vi "Ready Frequency Control for Sync.vi"(8 "error in (no error)":errorcluster, 11 "IED in":refnum<class "IED.lvclass">) -> (0 "error out":errorcluster, 3 "IED out":refnum<class "IED.lvclass">)   [LabVIEW 2015, in "IED Actor.lvlib" / "IED.lvclass"]
uses:
  IED.lvclass
  IED.lvclass/IED.ctl
  <vilib>/NI/Tools/Keyed Array/Map String.vi
  <vilib>/NI/Tools/String/Get Case Matching.vi
  <vilib>/Modbus/master/Modbus Master.lvclass
  <vilib>/NI/Tools/Keyed Array/Tools_KeyedArray.lvlib
  Utilities/Message Strings.llb/Message String Utilities.lvlib
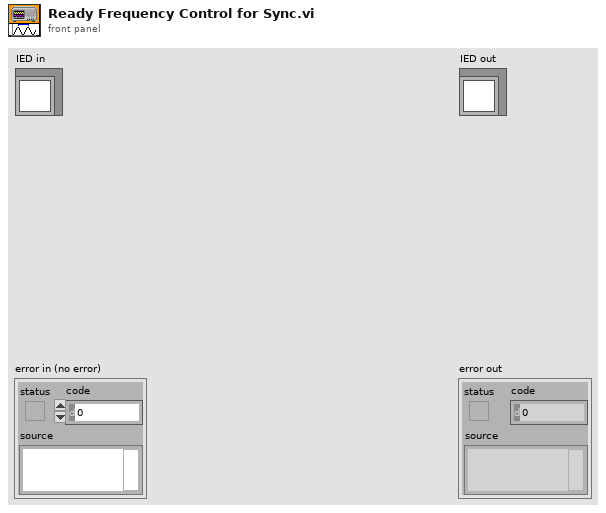
[diagram p1: front panel]
types:
  T1 = typedef "Tools_KeyedArray.lvlib/KeyedArray.ctl" = cluster{"keys":string[], "values":string[]}
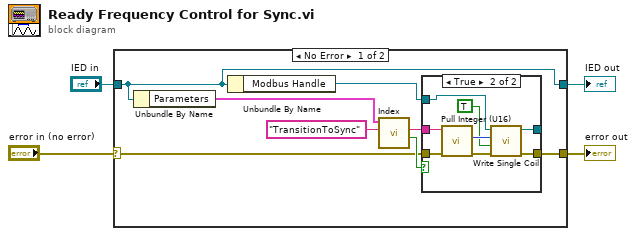
[diagram p0: block diagram]
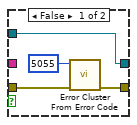
[diagram p2: hidden frame]
diagram:
  n1 = case shown="No Error" "error in (no error)" {
    selector: "error in (no error)" -> [w9 w26]
    tunnel: [w6 w26] -> w3
    tunnel: [w7 w25] -> w1
    tunnel: "IED in" -> [w7 w25]
    frame No Error {
      n2 = Unbundle By Name(w7) -> ("Parameters"=w12:T1)
      n3 = Unbundle By Name(w7) -> ("Modbus Handle"=w8:refnum<class "Modbus Master.lvclass">)
      n4 = call <vilib>:"Index.vi"("key"="TransitionToSync" ("Name"), "array in"=w12) -> ("valid key"=w11:bool, "value"=w10:string)  [unwired: 3 in, 1 out]
      n5 = case shown="True" w11 {
        tunnel: w10 -> [_ w24]
        tunnel: w8 -> [w13 w23]
        tunnel: w9 -> [w15 w22]
        tunnel: [w16 w19] -> w6
        tunnel: [w13 w18] -> _
        frame False {
          n6 = call <vilib>:"Error Cluster From Error Code.vi"("error in (no error)"=w15, "error code (0)"=5055) -> ("error out"=w16:errorcluster)  [unwired: 7 in]
        }
        frame True {
          n7 = call "Pull Integer (U16).vi"("error in (no error)"=w22, "String in"=w24) -> ("error out"=w21:errorcluster, "Integer out"=w20:u16)  [unwired: 7 in, 1 out]
          n8 = call-dynamic "Write Single Coil.vi"("error in (no error)"=w21, "coil value"=TRUE, "address"=w20, "Modbus master in"=w23) -> ("error out"=w19:errorcluster, "Modbus master out"=w18:refnum<class "Modbus Master.lvclass">)  [unwired: 6 in]
        }
      }
    }
    frame Error {
    }
  }
  "error out" <- w3
  "IED out" <- w1
